vi "Test 1.vi"() -> ()   [LabVIEW 2014]
uses:
  <vilib>/Aledyne-TSXperts/Arduino Compatible Compiler for LabVIEW/addons/test/test.lvlib
panel:
  out "result":u32
  out "error out":errorcluster
  in  "error in (no error)":errorcluster
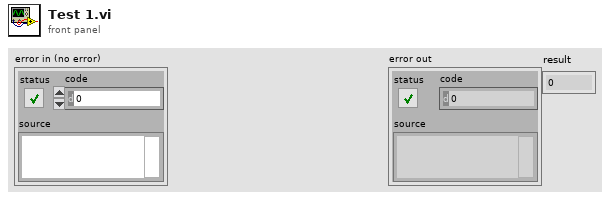
[diagram p1: front panel]
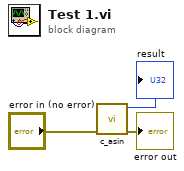
[diagram p0: block diagram]
diagram:
  n1 = call <vilib>:"c_asin.vi"("error in (no error)"="error in (no error)") -> ("error out"=→"error out":errorcluster, "result"=→"result":u32)  [unwired: 9 in]
